vi "VsEP-Options Dialog.vi"(0 "Options In":T1) -> (4 "Options OUt":T1, 8 "Canceled?":bool)   [LabVIEW 2020]
uses:
  Typedefs/VsEP-Hidden Params.ctl
  epl-vi-lib/Signal Synthesis VIs/Controls/Gate XCtl/Gate Control.xctl
panel:
  in  "Input sampling rate (Hz)":dbl
  in  "Output sampling rate (Hz)":dbl
  in  "Ramp (ms)":dbl
  in  "Delay (ms)":dbl
  in  "Attenuation (dB)":dbl
  in  "Cancel":bool
  in  "OK":bool
  # "Masking Noise"
  # "Note: the masking noise is on continuously, and delivered from the channel labeled \"Background\"\nin the Connection Manager."
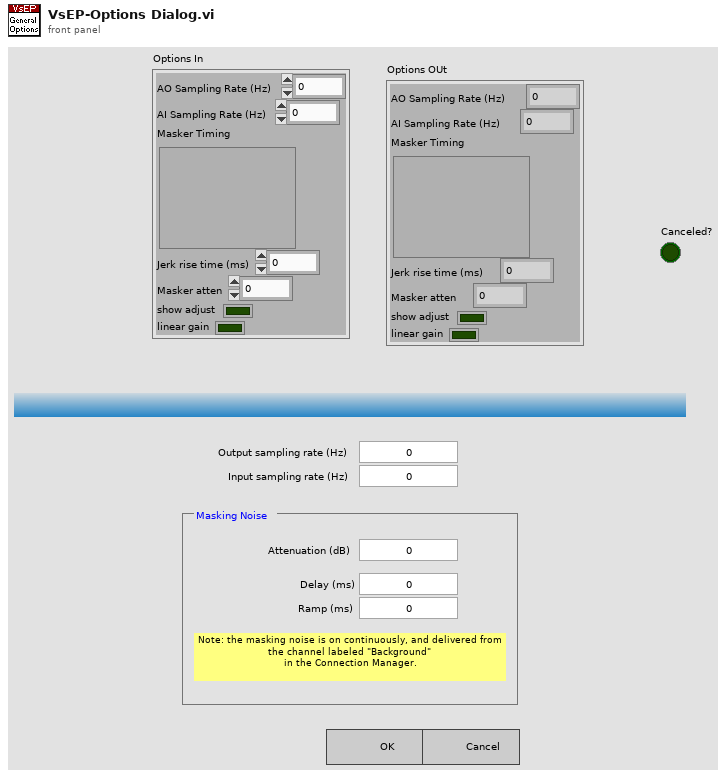
[diagram p1: front panel]
types:
  T1 = typedef "VsEP-Hidden Params.ctl" = cluster{"AO Sampling Rate (Hz)":dbl, "AI Sampling Rate (Hz)":dbl, "Masker Timing":cluster{"Active":bool, "Delay (ms)":dbl, "Width (ms)":dbl, "Ramp (ms)":dbl}, "Jerk rise time (ms)":dbl, "Masker atten":dbl, "show adjust":bool, "linear gain":bool}
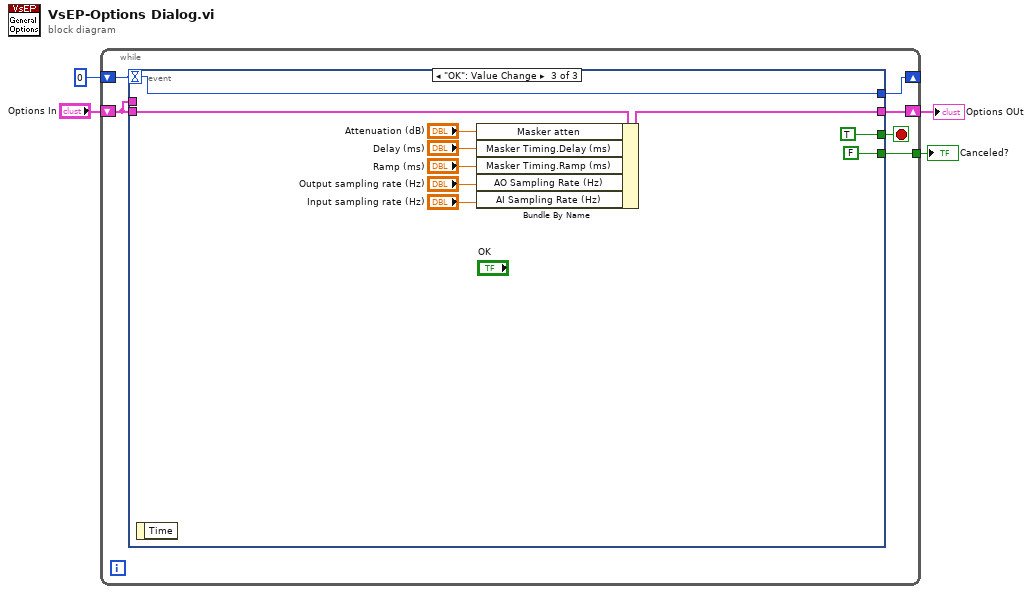
[diagram p0: block diagram]
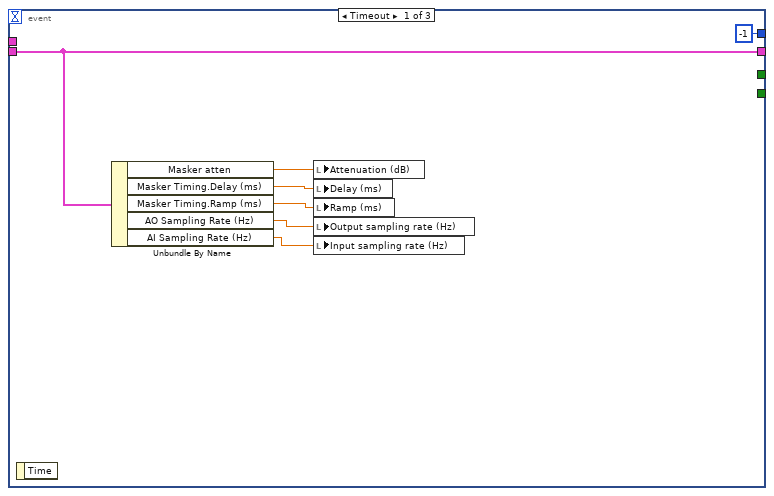
[diagram p2: hidden frame]
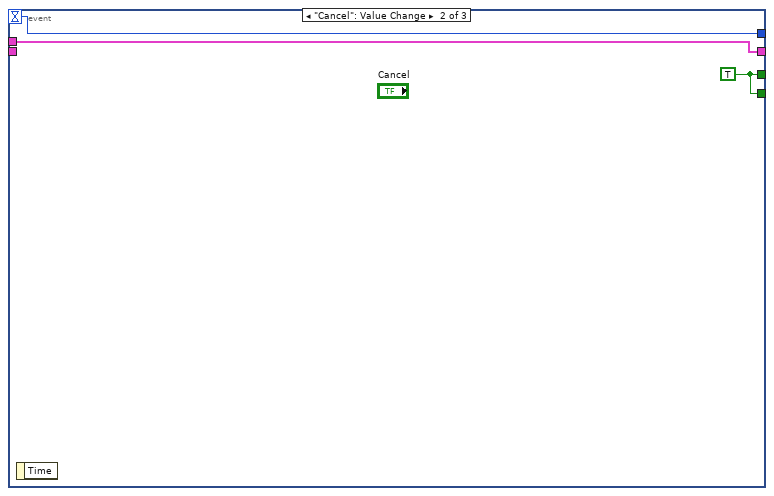
[diagram p3: hidden frame]
diagram:
  n1 = while {
    shift-right: [w9] -> _
    shift-left: 0 -> [w10]
    tunnel: [w6] -> w1
    shift-right: [w8] -> w2
    shift-left: "Options In" -> [w5]
    stop <- w7 stop-if-true
    n2 = event shown="[2] \"OK\": Value Change" {
      selector: _ -> [_ _ _]
      dyn-events: _ -> [_ _ _]
      timeout: w10 -> [_ w20 w29]
      tunnel: [-1 w20 w29] -> w9
      tunnel: w5 -> [w16 _ w30]
      tunnel: [w16 w18 w26] -> w8
      tunnel: [_ w19 TRUE] -> w7
      tunnel: [_ w19 FALSE] -> w6
      tunnel: w5 -> [_ w18 _]
      event Timeout {
        n3 = event-data() -> ()  [unwired: 1 in, 1 out]
        n4 = Unbundle By Name(w16) -> ("Masker atten"=w15:dbl, "Masker Timing.Delay (ms)"=w14:dbl, "Masker Timing.Ramp (ms)"=w13:dbl, "AO Sampling Rate (Hz)"=w12:dbl, "AI Sampling Rate (Hz)"=w11:dbl)
        n5 = local write "Attenuation (dB)"(w15) -> ()
        n6 = local write "Delay (ms)"(w14) -> ()
        n7 = local write "Ramp (ms)"(w13) -> ()
        n8 = local write "Output sampling rate (Hz)"(w12) -> ()
        n9 = local write "Input sampling rate (Hz)"(w11) -> ()
      }
      event "Cancel": Value Change {
        w19 = TRUE
        n10 = event-data() -> ()  [unwired: 1 in, 1 out]
      }
      event "OK": Value Change {
        n11 = event-data() -> ()  [unwired: 1 in, 1 out]
        n12 = Bundle By Name(cluster=w30, "Masker atten"="Attenuation (dB)", "Masker Timing.Delay (ms)"="Delay (ms)", "Masker Timing.Ramp (ms)"="Ramp (ms)", "AO Sampling Rate (Hz)"="Output sampling rate (Hz)", "AI Sampling Rate (Hz)"="Input sampling rate (Hz)") -> (w26:T1)
      }
    }
  }
  "Options OUt" <- w2
  "Canceled?" <- w1
